vi "fgv_Objectives.vi"(7 "Actions":T1(ring), 8 "error in (no error)":errorcluster, 10 "Objectives":string[](array[string]), 11 "Current Objective":string) -> (0 "error out":errorcluster, 2 "Objectives":string[](array[string]), 3 "Current Objective":string)   [LabVIEW 2020]
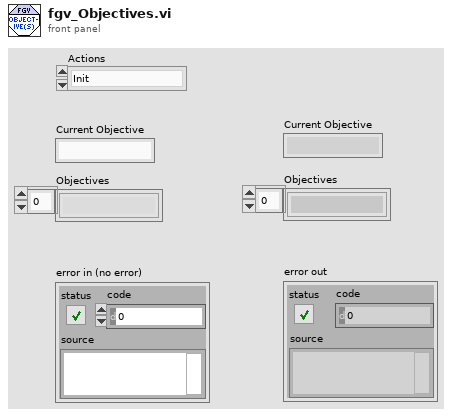
[diagram p1: front panel]
types:
  T1 = enum16{"Init", "Update Objectives", "Update Current Objective", "Read", "Clear"}
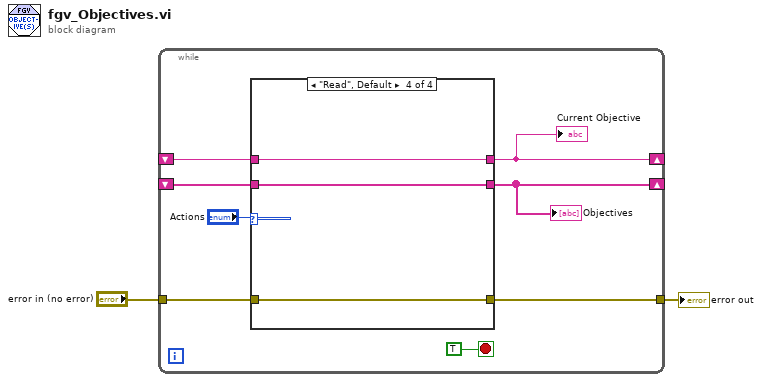
[diagram p0: block diagram]
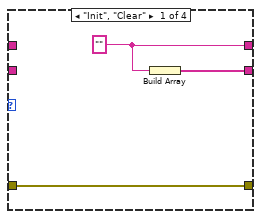
[diagram p2: hidden frame]
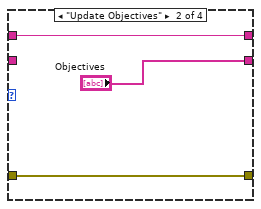
[diagram p3: hidden frame]
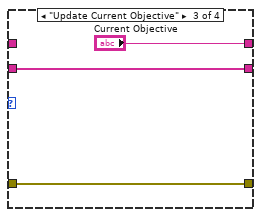
[diagram p4: hidden frame]
diagram:
  n1 = while {
    tunnel: "error in (no error)" -> [w8]
    shift-right: [w7] -> _
    shift-left: _ -> [w6]
    shift-right: [w5] -> _
    shift-left: _ -> [w4]
    tunnel: [w3] -> w1
    stop <- TRUE stop-if-true
    n2 = case shown="\"Read\", Default" "Actions" {
      tunnel: w8 -> [w11 w14 w17 w20]
      tunnel: [w13 w16 "Current Objective" w22] -> w7
      tunnel: w6 -> [_ w16 _ w22]
      tunnel: [w12 "Objectives" w19 w21] -> w5
      tunnel: w4 -> [_ _ w19 w21]
      tunnel: [w11 w14 w17 w20] -> w3
      frame "Init", "Clear" {
        w13 = ""
        n3 = Build Array(w13) -> (w12:string[])
      }
      frame "Update Objectives" {
      }
      frame "Update Current Objective" {
      }
      frame "Read", Default {
      }
    }
    "Current Objective" <- w7
    "Objectives" <- w5
  }
  "error out" <- w1
